vi "SimplePackUnpack.vi"() -> ()   [LabVIEW 2019]
uses:
  <vilib>/gRPC/LabVIEW gRPC Library/Server API/typeDefs/Message Metadata.ctl
  <vilib>/gRPC/LabVIEW gRPC Library/Server API/typeDefs/Message Element Metadata.ctl
  <vilib>/gRPC/LabVIEW gRPC Library/Server API/typeDefs/Message Element Type.ctl
  7fd04eb5-0132-428e-93dc-a7bf2da436d2.vi
  487e9c1f-f261-4604-8385-308564aa59d5.vi
  <vilib>/gRPC/LabVIEW gRPC Library/Server API/Server/Get Server DLL Path.vi
  <vilib>/gRPC/LabVIEW gRPC Library/gprc-lvsupport-release.lvlib
panel:
  out "error out":errorcluster
  out "Numeric":i32
  out "x = y?":bool
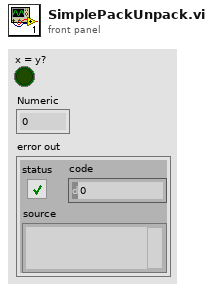
[diagram p1: front panel]
types:
  T1 = typedef "gprc-lvsupport-release.lvlib/Message Metadata.ctl" = cluster{"Version":i32, "Name":string, "Type Url":string, "Elements":T2[]}
  T2 = typedef "gprc-lvsupport-release.lvlib/Message Element Metadata.ctl" = cluster{"Embedded Message Name":string, "Protobuf Index":i32, "MessageElementType":T3, "Repeated":bool}
  T3 = typedef "gprc-lvsupport-release.lvlib/Message Element Type.ctl" = enum32{"Int32Value", "FloatValue", "DoubleValue", "BoolValue", "StringValue", "MessageValue", "Int64Value", "UInt32Value", "UInt64Value", "EnumValue", "Bytes", "Fixed64", "Fixed32", "SFixed64", "SFixed32", "SInt64", "SInt32"}
  T4 = typedef "gprc-lvsupport-release.lvlib/grpcId.ctl" = u64
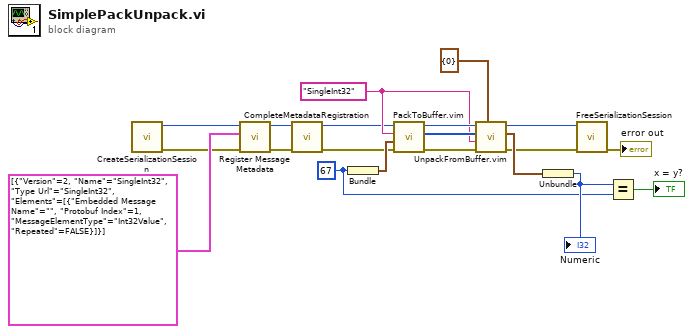
[diagram p0: block diagram]
diagram:
  w10 = 67
  w13 = "SingleInt32" ("Message Type")
  n1 = call <vilib>:"CreateSerializationSession.vi"() -> ("error out"=w6:errorcluster, "Serialization Session ID"=w20:T4)  [unwired: 10 in]
  n2 = call <vilib>:"Register Message Metadata.vi"("error in (no error)"=w6, "Messages"=T1[] [{"Version"=2, "Name"="SingleInt32", "Type Url"="SingleInt32", "Elements"=[{"Embedded Message Name"="", "Protobuf Index"=1, "MessageElementType"=enum."Int32Value", "Repeated"=FALSE}]}], "gRPCid"=w20) -> ("error out"=w5:errorcluster, "gRPCid"=w8:T4)  [unwired: 7 in]
  n3 = call <vilib>:"CompleteMetadataRegistration.vi"("error in (no error)"=w5, "gRPC ID"=w8) -> ("error out"=w4:errorcluster, "gRPC ID Out"=w7:T4)  [unwired: 8 in]
  n4 = Bundle(w10) -> (w18:cluster{i32})  [unwired: 1 in]
  n5 = call "PackToBuffer.vim"("error in (no error)"=w4, "Data To Pack"=w18, "Message Type"=w13, "gRPCid in"=w7) -> ("error out"=w3:errorcluster, "Buffer"=w14:u8[], "gRPCid out"=w17:u64)  [unwired: 5 in]
  n6 = call "UnpackFromBuffer.vim"("Data Type"=cluster{i32} {0}, "error in (no error)"=w3, "Message Type"=w13, "Buffer"=w14, "gRPCid in"=w17) -> ("error out"=w2:errorcluster, "Unpacked Value"=w12:cluster{i32}, "gRPCid"=w16:u64)  [unwired: 4 in]
  n7 = Unbundle(w12) -> (w11:i32)
  "Numeric" <- w11
  n8 = call <vilib>:"FreeSerializationSession.vi"("error in (no error)"=w2, "Serialization Session ID"=w16) -> ("error out"=→"error out":errorcluster)  [unwired: 9 in]
  n9 = Equal?(x=w11, y=w10) -> (x = y?=→"x = y?":bool)
